vi "StopCapture.vi"(8 "error in (no error)":errorcluster, 11 "Hamamatsu_Camera in":refnum<class "Hamamatsu_Camera.lvclass">) -> (0 "error out":errorcluster, 3 "Hamamatsu_Camera out":refnum<class "Hamamatsu_Camera.lvclass">)   [LabVIEW 2023, in "Hamamatsu_Camera.lvlib" / "Hamamatsu_Camera.lvclass"]
uses:
  Hamamatsu_Camera.lvclass
  C:/Program Files/National Instruments/LabVIEW 2023/vi.lib/ActorFramework/Actor/Actor.lvclass
  Hamamatsu_Camera.lvclass/Hamamatsu_Camera.ctl
  <vilib>/ActorFramework/Actor/Actor.lvclass/Actor.ctl
  <vilib>/ActorFramework/Message Enqueuer/Message Enqueuer.lvclass/Message Enqueuer.ctl
  <vilib>/ActorFramework/Message Enqueuer/Enqueue.vi
  Interfaces/AbstractInstrumentClasses/Cameras_LV/CameraComm Messages/Capture Stopped Msg/Capture Stopped Msg.lvclass
  C:/Program Files/National Instruments/LabVIEW 2023/vi.lib/ActorFramework/Message/Message.lvclass
  <vilib>/ActorFramework/Message Priority Queue/Priority Enqueue.vi
  <vilib>/ActorFramework/Actor/Actor.lvclass
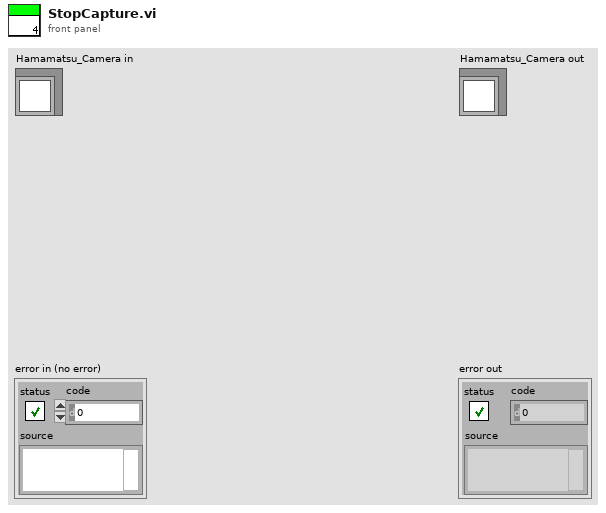
[diagram p1: front panel]
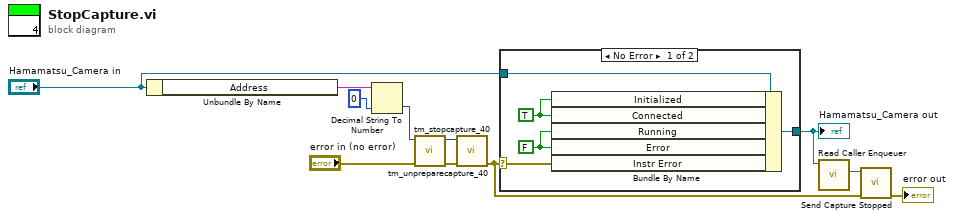
[diagram p0: block diagram]
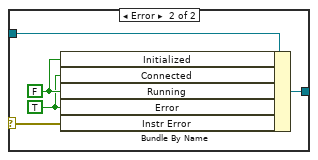
[diagram p2: hidden frame]
diagram:
  n1 = Unbundle By Name("Hamamatsu_Camera in") -> ("Address"=w11:string)
  n2 = Decimal String To Number(string=w11, default (0L)=u32 0 ("default (0 I32)")) -> (number=w9:u32)  [unwired: 1 in, 1 out]
  n3 = call "tm_stopcapture_40.vi"("error in (no error)"="error in (no error)", "Handle in"=w9) -> ("error out"=w4:errorcluster, "Handle out"=w5:u32)  [unwired: 8 in]
  n4 = call "tm_unpreparecapture_40.vi"("error in (no error)"=w4, "Handle in"=w5) -> ("error out"=w1:errorcluster)  [unwired: 8 in, 1 out]
  n5 = case shown="No Error" w1 {
    selector: w1 -> [w13 w18]
    tunnel: "Hamamatsu_Camera in" -> [w16 w21]
    tunnel: [w14 w19] -> w2
    frame No Error {
      w12 = TRUE ("InstrumentData.CurrentState.Connected")
      w15 = FALSE ("InstrumentData.CurrentState.Initialized")
      n6 = Bundle By Name(cluster=w16, "Initialized"=w12, "Connected"=w12, "Running"=w15, "Error"=w15, "Instr Error"=w13) -> (w14:refnum<class "Hamamatsu_Camera.lvclass">)
    }
    frame Error {
      w17 = TRUE ("InstrumentData.CurrentState.Connected")
      w20 = FALSE ("InstrumentData.CurrentState.Initialized")
      n7 = Bundle By Name(cluster=w21, "Initialized"=w20, "Connected"=w17, "Running"=w20, "Error"=w17, "Instr Error"=w18) -> (w19:refnum<class "Hamamatsu_Camera.lvclass">)
    }
  }
  "Hamamatsu_Camera out" <- w2
  n8 = call <vilib>:"Read Caller Enqueuer.vi"("Actor"=w2) -> ("Caller Enqueuer"=w7:refnum<class "Message Enqueuer.lvclass">)  [unwired: 10 in]
  n9 = call "Send Capture Stopped.vi"("error in (no error)"=w1, "Message Enqueuer"=w7) -> ("error out"=→"error out":errorcluster)  [unwired: 8 in, 1 out]
